vi "CreateLogFile.vi"(5 "Stop Time":timestamp[](array[timestamp]), 7 "Start Time":timestamp[](array[timestamp]), 9 "Log?":bool, 10 "HAL Config":T1[](array[typedef]), 11 "ACQ Queues":refnum<queue>[](array[refnum])) -> ()   [LabVIEW 2014]
uses:
  APIs/Data Queue/Acquisition Data 1 Sample Cluster.ctl
  TypeDefs/HAL Config Data.ctl
  APIs/Data Queue/WINFAS 2 Data Queue.lvlib
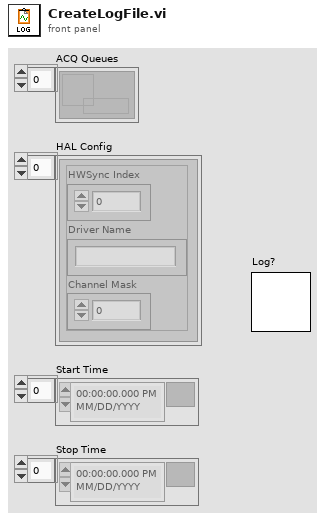
[diagram p1: front panel]
types:
  T1 = typedef "HAL Config Data.ctl" = cluster{"HWSync Index":u32, "Driver Name":string, "Channel Mask":u64}
  T2 = enum16{"open", "replace", "create", "open or create", "replace or create", "replace or create with confirmation"}
  T3 = typedef "WINFAS 2 Data Queue.lvlib/Acquisition Data 1 Sample Cluster.ctl" = cluster{"TDX":sgl[], "Encoder":sgl}
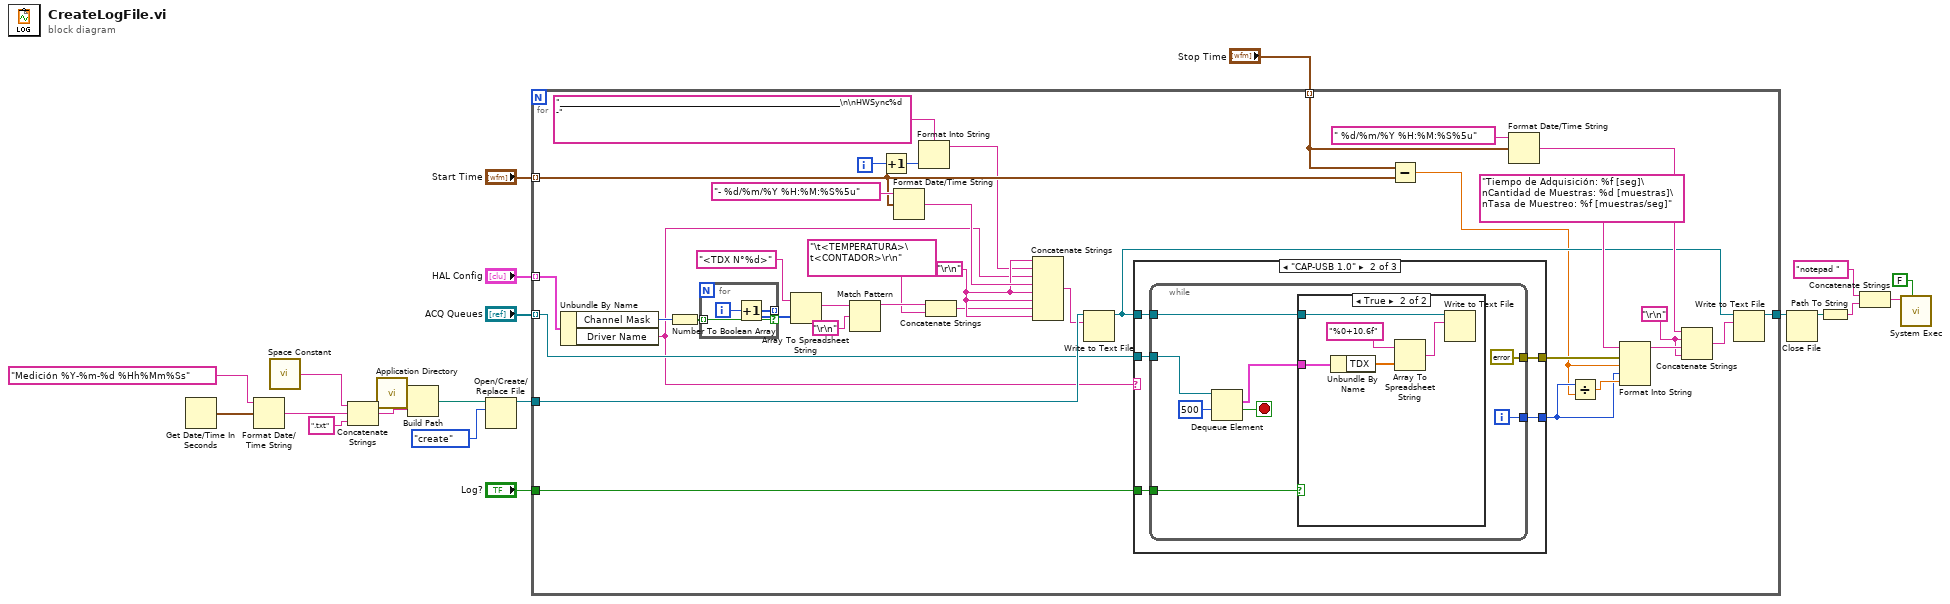
[diagram p0: block diagram]
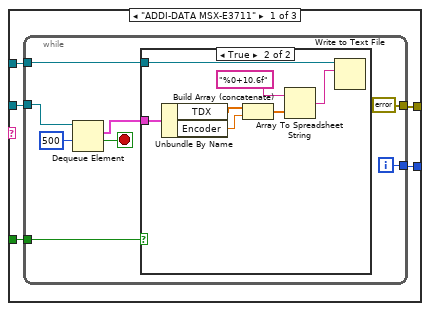
[diagram p2: hidden frame]
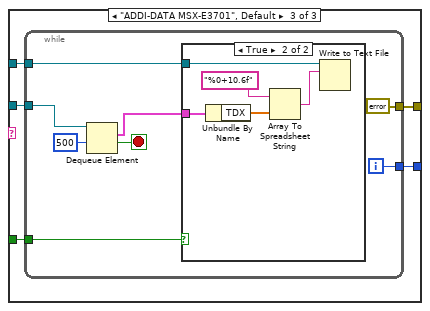
[diagram p5: hidden frame]
diagram:
  n1 = Get Date/Time In Seconds() -> (seconds since 1Jan1904=w6:timestamp)
  n2 = Format Date/Time String(time format string (%c)="Medición %Y-%m-%d %Hh%Mm%Ss" ("string"), seconds (now)=w6) -> (date/time string=w7:string)  [unwired: 1 in]
  n3 = call <vilib>:"Space Constant.vi"() -> ("String"=w13:string)
  n4 = Concatenate Strings(w13, w7, ".txt" ("string")) -> (w9:string)
  n5 = call <vilib>:"Application Directory.vi"() -> ("Application Directory"=w12:path)
  n6 = Build Path(base path=w12, name or relative path=w9) -> (appended path=w11:path)
  n7 = Open/Create/Replace File(file path (use dialog)=w11, operation (0:open)=T2."create") -> (refnum out=w5:refnum<file>)  [unwired: 4 in, 2 out]
  n8 = for {
    tunnel: "HAL Config" -> [w51] mode=indexing
    tunnel: "Stop Time" -> [w33] mode=indexing
    tunnel: "Start Time" -> [w32] mode=indexing
    tunnel: w5 -> [w41]
    tunnel: [w42] -> w4
    tunnel: "ACQ Queues" -> [w31] mode=indexing
    tunnel: "Log?" -> [w22]
    i -> [w34]
    w39 = "\r\n"
    w38 = "\r\n"
    n9 = Unbundle By Name(w51) -> ("Channel Mask"=w56:u64, "Driver Name"=w30:string)
    n10 = Number To Boolean Array(number=w56) -> (Boolean array=w55:bool[])
    n11 = for {
      tunnel: w55 -> [w116] mode=indexing
      tunnel: [w114] -> w54 mode=indexing if=w116
      i -> [w115]
      n12 = Increment(x=w115) -> (x+1=w114:i32)
    }
    n13 = Array To Spreadsheet String(array=w54, 3:"<TDX N°%d>" ("format string")) -> (spreadsheet string=w24:string)  [unwired: 1 in]
    n14 = Match Pattern(string=w24, regular expression="\r\n") -> (before substring=w28:string)  [unwired: 1 in, 3 out]
    n15 = Increment(x=w34) -> (x+1=w50:i32)
    n16 = Format Date/Time String(time format string (%c)="- %d/%m/%Y %H:%M:%S%5u" ("string"), seconds (now)=w32) -> (date/time string=w57:string)  [unwired: 1 in]
    n17 = Format Into String(format string="______________________________________________________________________\n\nHWSync%d -", w50) -> (resulting string=w29:string)  [unwired: 2 in, 1 out]
    n18 = Concatenate Strings(w28, "\t<TEMPERATURA>\t<CONTADOR>\r\n" ("format string")) -> (w25:string)
    n19 = Concatenate Strings(w38, w29, w30, w57, w38, w38, w25, w38) -> (w40:string)
    n20 = Write to Text File(file (use dialog)=w41, text=w40) -> (refnum out=w37:refnum<file>)  [unwired: 2 in, 2 out]
    n21 = case shown="\"CAP-USB 1.0\"" w30 {
      tunnel: w37 -> [w61 w82 w100]
      tunnel: [w60 w81 w99] -> w36
      tunnel: [w59 w80 w98] -> w35
      tunnel: w31 -> [w62 w79 w97]
      tunnel: w22 -> [w58 w78 w96]
      frame "ADDI-DATA MSX-E3711" {
        n22 = while {
          tunnel: w62 -> [w68]
          tunnel: w61 -> [w70]
          tunnel: [errorcluster {"status"=FALSE, "code"=0, "source"=""} ("error constant")] -> w60
          tunnel: [w64] -> w59
          tunnel: w58 -> [w63]
          i -> [w64]
          stop <- w65 stop-if-true
          n23 = Dequeue Element(queue=w68, timeout in ms (-1)=500) -> (element=w67:T3, timed out?=w65:bool)  [unwired: 1 in, 2 out]
          n24 = case shown="True" w63 {
            tunnel: w70 -> [_ w75]
            tunnel: w67 -> [_ w74]
            frame False {
            }
            frame True {
              n25 = Unbundle By Name(w74) -> ("TDX"=w72:sgl[], "Encoder"=w73:sgl)
              n26 = Build Array (concatenate)(w72, w73) -> (w71:sgl[])
              n27 = Array To Spreadsheet String(array=w71, 3:"%0+10.6f" ("format string")) -> (spreadsheet string=w76:string)  [unwired: 1 in]
              n28 = Write to Text File(file (use dialog)=w75, text=w76) -> ()  [unwired: 2 in, 3 out]
            }
          }
        }
      }
      frame "CAP-USB 1.0" {
        n29 = while {
          tunnel: w79 -> [w88]
          tunnel: w82 -> [w90]
          tunnel: [errorcluster {"status"=FALSE, "code"=0, "source"=""} ("error constant")] -> w81
          tunnel: [w84] -> w80
          tunnel: w78 -> [w83]
          i -> [w84]
          stop <- w85 stop-if-true
          n30 = Dequeue Element(queue=w88, timeout in ms (-1)=500) -> (element=w87:T3, timed out?=w85:bool)  [unwired: 1 in, 2 out]
          n31 = case shown="True" w83 {
            tunnel: w90 -> [_ w92]
            tunnel: w87 -> [_ w91]
            frame False {
            }
            frame True {
              n32 = Unbundle By Name(w91) -> ("TDX"=w95:sgl[])
              n33 = Array To Spreadsheet String(array=w95, 3:"%0+10.6f" ("format string")) -> (spreadsheet string=w93:string)  [unwired: 1 in]
              n34 = Write to Text File(file (use dialog)=w92, text=w93) -> ()  [unwired: 2 in, 3 out]
            }
          }
        }
      }
      frame "ADDI-DATA MSX-E3701", Default {
        n35 = while {
          tunnel: w97 -> [w106]
          tunnel: w100 -> [w108]
          tunnel: [errorcluster {"status"=FALSE, "code"=0, "source"=""} ("error constant")] -> w99
          tunnel: [w102] -> w98
          tunnel: w96 -> [w101]
          i -> [w102]
          stop <- w103 stop-if-true
          n36 = Dequeue Element(queue=w106, timeout in ms (-1)=500) -> (element=w105:T3, timed out?=w103:bool)  [unwired: 1 in, 2 out]
          n37 = case shown="True" w101 {
            tunnel: w108 -> [_ w110]
            tunnel: w105 -> [_ w109]
            frame False {
            }
            frame True {
              n38 = Unbundle By Name(w109) -> ("TDX"=w113:sgl[])
              n39 = Array To Spreadsheet String(array=w113, 3:"%0+10.6f" ("format string")) -> (spreadsheet string=w111:string)  [unwired: 1 in]
              n40 = Write to Text File(file (use dialog)=w110, text=w111) -> ()  [unwired: 2 in, 3 out]
            }
          }
        }
      }
    }
    n41 = Subtract(x=w33, y=w32) -> (x-y=w23:dbl)
    n42 = Format Date/Time String(time format string (%c)=" %d/%m/%Y %H:%M:%S%5u" ("string"), seconds (now)=w33) -> (date/time string=w43:string)  [unwired: 1 in]
    n43 = Divide(x=w35, y=w23) -> (x/y=w46:dbl)
    n44 = Format Into String(format string="Tiempo de Adquisición: %f [seg]\nCantidad de Muestras: %d [muestras]\nTasa de Muestreo: %f [muestras/seg]" ("string"), error in=w36, w23, w35, w46) -> (resulting string=w48:string)  [unwired: 1 in, 1 out]
    n45 = Concatenate Strings(w43, w39, w48, w39) -> (w44:string)
    n46 = Write to Text File(file (use dialog)=w37, text=w44) -> (refnum out=w42:refnum<file>)  [unwired: 2 in, 2 out]
  }
  n47 = Close File(refnum=w4) -> (path=w3:path)  [unwired: 1 in, 1 out]
  n48 = Path To String(path=w3) -> (string=w16:string)
  n49 = Concatenate Strings("notepad ", w16) -> (w18:string)
  n50 = call <vilib>:"System Exec.vi"("wait until completion? (T)"=FALSE, "command line"=w18) -> ()  [unwired: 6 in, 4 out]
